vi "Untitled 1.vi"() -> ()   [LabVIEW 2011]
uses:
  <vilib>/DAQmx/read.llb/DAQmx Read (Digital Bool 1Line 1Point).vi
  <vilib>/DAQmx/create/channels.llb/DAQmx Create Channel (DI-Digital Input).vi
  <vilib>/DAQmx/miscellaneous.llb/DAQmx Fill In Error Info.vi
panel:
  out "Numeric":i32
  out "Boolean":bool
  out "x/y":i32
  in  "STOP":bool
  in  "Vasil":bool
  in  "Push":bool
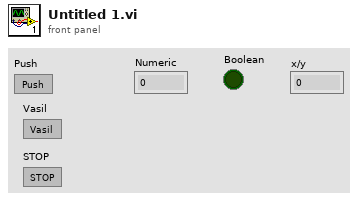
[diagram p1: front panel]
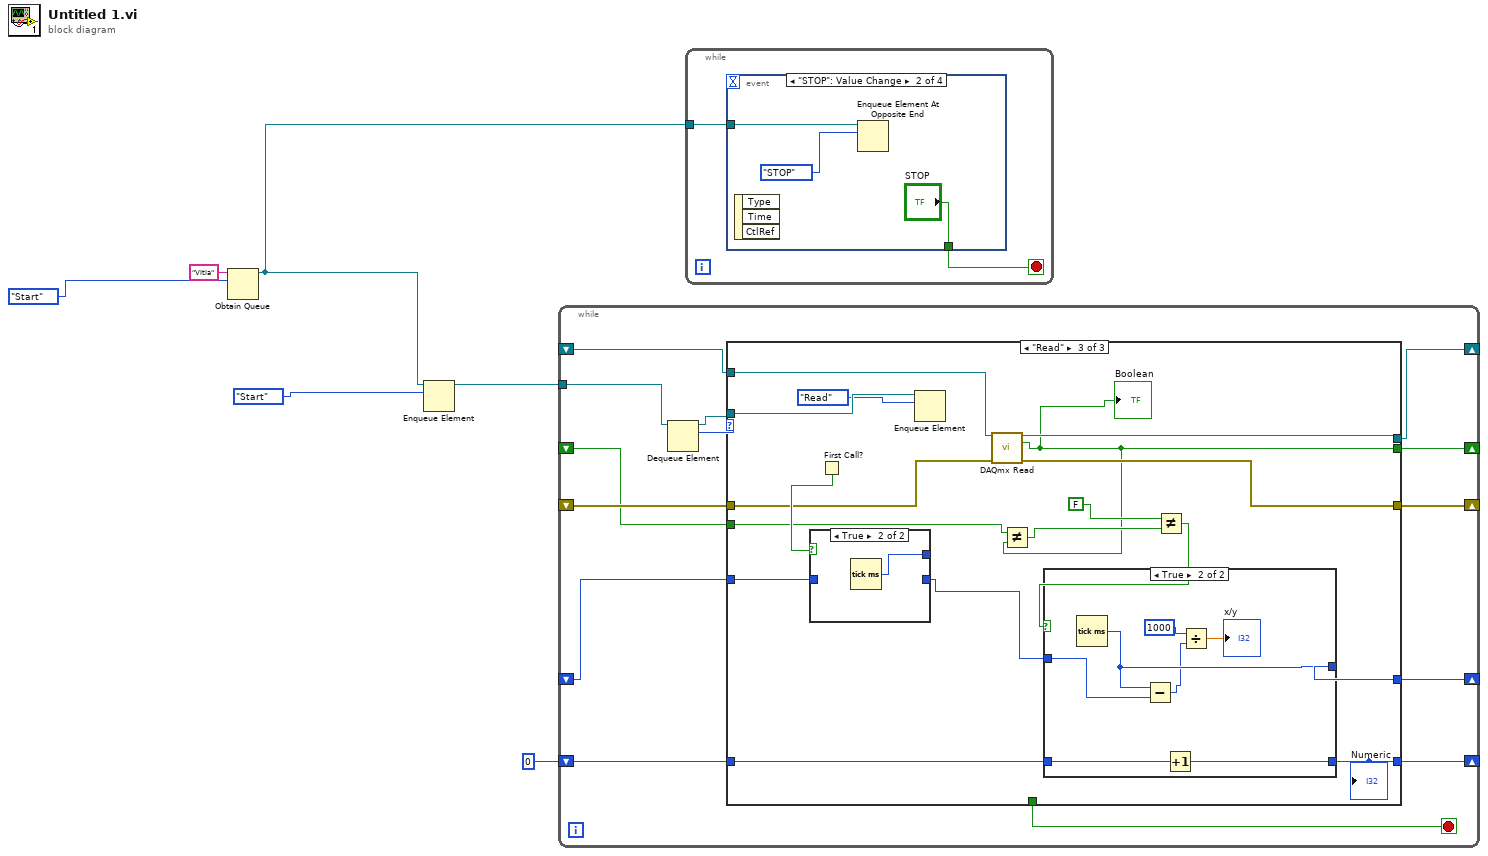
[diagram p0: block diagram]
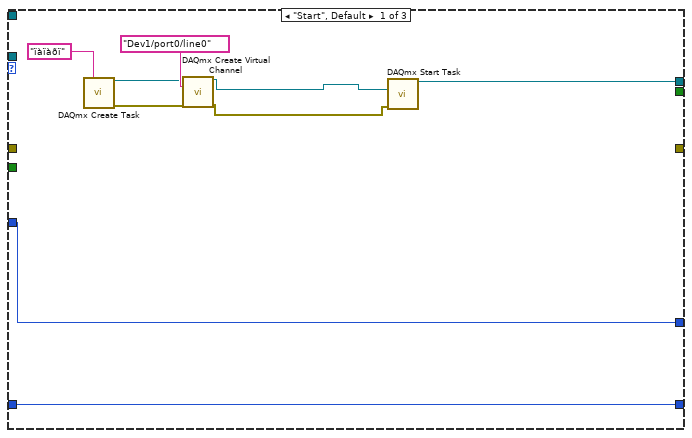
[diagram p2: hidden frame]
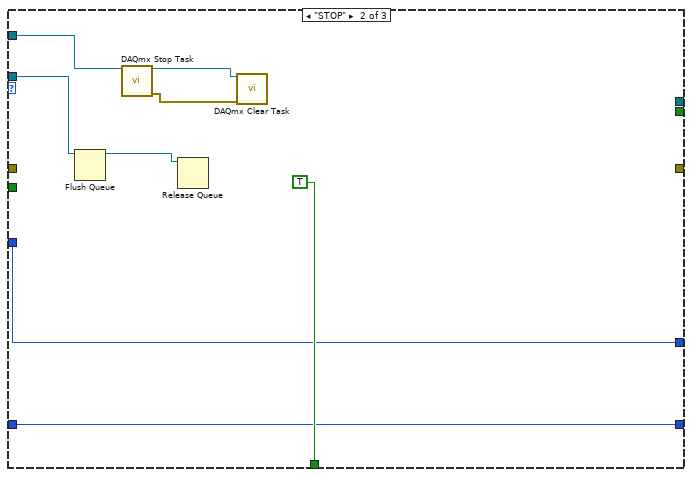
[diagram p3: hidden frame]
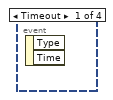
[diagram p6: hidden frame]
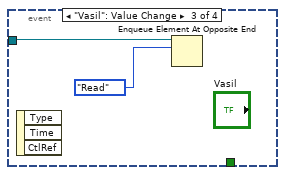
[diagram p7: hidden frame]
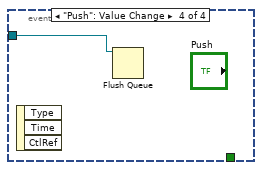
[diagram p8: hidden frame]
diagram:
  n1 = Obtain Queue(name (unnamed)="Vitia", element data type=enum16{"Start", "STOP", "Read"}."Start" ("Enum")) -> (queue out=w4:refnum<queue>)  [unwired: 3 in, 2 out]
  n2 = Enqueue Element(queue=w4, element=enum16{"Start", "STOP", "Read"}."Start" ("Enum")) -> (queue out=w2:refnum<queue>)  [unwired: 2 in, 2 out]
  n3 = while {
    tunnel: w2 -> [w20]
    shift-right: [w15] -> _
    shift-left: _ -> [w14]
    shift-right: [w9] -> _
    shift-left: _ -> [w16]
    shift-right: [w11] -> _
    shift-left: _ -> [w10]
    shift-right: [w12] -> _
    shift-left: _ -> [w13]
    shift-right: [w7] -> _
    shift-left: 0 -> [w8]
    stop <- w17 stop-if-true
    n4 = Dequeue Element(queue=w20) -> (queue out=w18:refnum<queue>, element=w19:enum16{"Start", "STOP", "Read"})  [unwired: 2 in, 2 out]
    n5 = case shown="\"Read\"" w19 {
      tunnel: w14 -> [_ w37 w48]
      tunnel: w18 -> [_ w34 w51]
      tunnel: [_ TRUE _] -> w17
      tunnel: [w25 _ w49] -> w15
      tunnel: w16 -> [w22 w31 w53]
      tunnel: w13 -> [_ _ w47]
      tunnel: [_ _ w46] -> w12
      tunnel: [_ _ w40] -> w11
      tunnel: w10 -> [_ _ w44]
      tunnel: [w22 w31 w41] -> w9
      tunnel: w8 -> [w21 w30 w39]
      tunnel: [w21 w30 w38] -> w7
      frame "Start", Default {
        n6 = call <vilib>:"DAQmx Create Task.vi"("new task name"="ïàïàðï") -> ("task out"=w26:refnum<k21>, "error out"=w28:errorcluster)  [unwired: 13 in]
        n7 = call-poly <vilib>:"DAQmx Create Virtual Channel.vi"("task in"=w26, "lines"=tag "Dev1/port0/line0", "error in"=w28) -> ("task out"=w24:refnum<k21>, "error out"=w23:errorcluster)  [unwired: 11 in]
        n8 = call <vilib>:"DAQmx Start Task.vi"("task/channels in"=w24, "error in"=w23) -> ("task out"=w25:refnum<k21>)  [unwired: 12 in, 1 out]
      }
      frame "STOP" {
        n9 = Flush Queue(queue=w34) -> (queue out=w33:refnum<queue>)  [unwired: 1 in, 2 out]
        n10 = call <vilib>:"DAQmx Stop Task.vi"("task/channels in"=w37) -> ("task out"=w36:refnum<k21>, "error out"=w35:errorcluster)  [unwired: 13 in]
        n11 = Release Queue(queue=w33) -> ()  [unwired: 2 in, 3 out]
        n12 = call <vilib>:"DAQmx Clear Task.vi"("task in"=w36, "error in"=w35) -> ()  [unwired: 13 in, 1 out]
      }
      frame "Read" {
        n13 = First Call?() -> (First Call?: T/F=w54:bool)
        n14 = case shown="True" w54 {
          tunnel: w53 -> [w55 _]
          tunnel: [w55 _] -> w52
          tunnel: [_ w56] -> _
          frame False {
          }
          frame True {
            n15 = Tick Count (ms)() -> (millisecond timer value=w56:u32)
          }
        }
        n16 = Enqueue Element(queue=w51, element=enum16{"Start", "STOP", "Read"}."Read" ("Enum")) -> ()  [unwired: 2 in, 3 out]
        n17 = call-poly <vilib>:"DAQmx Read.vi"("task/channels in"=w48, "error in"=w47) -> ("task out"=w49:refnum<k21>, "data"=w40:bool, "error out"=w46:errorcluster)  [unwired: 11 in]
        "Boolean" <- w40
        n18 = Not Equal?(x=w44, y=w40) -> (x != y?=w43:bool)
        n19 = Not Equal?(x=FALSE, y=w43) -> (x != y?=w42:bool)
        n20 = case shown="True" w42 {
          tunnel: w52 -> [w58 w61]
          tunnel: [w58 w63] -> w41
          tunnel: w39 -> [w57 w60]
          tunnel: [w57 w59] -> w38
          frame False {
          }
          frame True {
            n21 = Tick Count (ms)() -> (millisecond timer value=w63:u32)
            n22 = Subtract(x=w63, y=w61) -> (x-y=w62:u32)
            n23 = Increment(x=w60) -> (x+1=w59:i32)
            n24 = Divide(x=1000, y=w62) -> (x/y=→"x/y":dbl)
          }
        }
        "Numeric" <- w38
      }
    }
  }
  n25 = while {
    tunnel: w4 -> [w66]
    stop <- w67 stop-if-true
    n26 = event shown="[1] \"STOP\": Value Change" {
      selector: _ -> [_ _ _ _]
      dyn-events: _ -> [_ _ _ _]
      timeout: _ -> [_ _ _ _]
      tunnel: [_ "STOP" _ _] -> w67
      tunnel: w66 -> [_ w68 w71 w73]
      event Timeout {
        n27 = event-data() -> ()  [unwired: 1 in, 2 out]
      }
      event "STOP": Value Change {
        n28 = event-data() -> ()  [unwired: 1 in, 3 out]
        n29 = Enqueue Element At Opposite End(queue=w68, element=enum16{"Start", "STOP", "Read"}."STOP" ("Enum")) -> ()  [unwired: 2 in, 3 out]
      }
      event "Vasil": Value Change {
        n30 = event-data() -> ()  [unwired: 1 in, 3 out]
        n31 = Enqueue Element At Opposite End(queue=w71, element=enum16{"Start", "STOP", "Read"}."Read" ("Enum")) -> ()  [unwired: 2 in, 3 out]
      }
      event "Push": Value Change {
        n32 = event-data() -> ()  [unwired: 1 in, 3 out]
        n33 = Flush Queue(queue=w73) -> ()  [unwired: 1 in, 3 out]
      }
    }
  }
